vi "plc read string.vi"(8 "error in":errorcluster, 10 "Timeout (ms)":i32=1000, 11 "addr,tag":T1 {"DataSocket Reference"."OnStatusUpdated" format="%.0x"; "DataSocket Reference"."OnDataUpdated" format="%.0x"}) -> (0 "error out":errorcluster, 3 "Data":string)   [LabVIEW 2018]
uses:
  05.UserVI's/type defs/plc path and tag.ctl
  <vilib>/Platform/dataskt.llb/DataSocket Reference Type.ctl
  <vilib>/ethernetip/ethernetip.llb/EthernetIP Tag Read STRING.vi
  <vilib>/ethernetip/ethernetip.llb/EthernetIP Tag Read DINT.vi
  <vilib>/ethernetip/ethernetip.lvlib
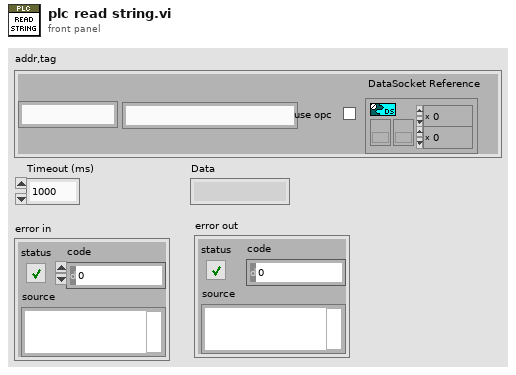
[diagram p1: front panel]
types:
  T1 = typedef "plc path and tag.ctl" = cluster{"Tag Name":string, "Network Path":string, "use opc":bool, "DataSocket Reference":T2}
  T2 = typedef "DataSocket Reference Type.ctl" = cluster{"CWDSLib._DCWDataSocket":refnum<k7>, "CWDSLib._DCWData":refnum<k7>, "OnDataUpdated":u32, "OnStatusUpdated":u32}
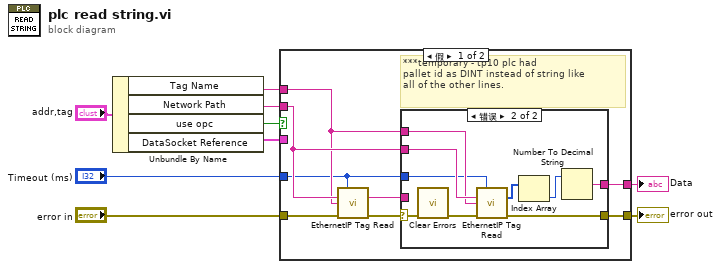
[diagram p0: block diagram]
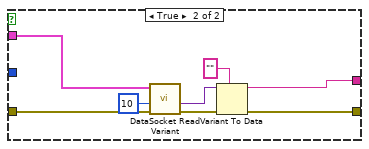
[diagram p3: hidden frame]
diagram:
  n1 = Unbundle By Name("addr,tag") -> ("Tag Name"=w4:string, "Network Path"=w5:string, "use opc"=w2:bool, "DataSocket Reference"=w1:T2)
  n2 = case shown="假" w2 {
    tunnel: "error in" -> [w17 w34]
    tunnel: [w14 w32] -> w7
    tunnel: [w13 w29] -> w6
    tunnel: w5 -> [w12 _]
    tunnel: w4 -> [w11 _]
    tunnel: "Timeout (ms)" -> [w10 _]
    tunnel: w1 -> [_ w35]
    frame False {
      # "***temporary - tp10 plc had\npallet id as DINT instead of string like\nall of the other lines."
      n3 = call-poly <vilib>:"EthernetIP Tag Read.vi"("Timeout (ms)"=w10, "Network Path"=w12, "Tag Name"=w11, "error in"=w17) -> ("Data"=w15:string, "error out"=w16:errorcluster)  [unwired: 9 in, 1 out]
      n4 = case shown="错误" w16 {
        selector: w16 -> [w18 w22]
        tunnel: [w19 w25] -> w13
        tunnel: w15 -> [w19 _]
        tunnel: w12 -> [_ w28]
        tunnel: w11 -> [_ w27]
        tunnel: [w18 w23] -> w14
        tunnel: w10 -> [_ w20]
        frame No Error {
        }
        frame Error {
          n5 = call <vilib>:"Clear Errors.vi"("error in (no error)"=w22) -> ("error out"=w21:errorcluster)  [unwired: 5 in, 1 out]
          n6 = call-poly <vilib>:"EthernetIP Tag Read.vi"("Timeout (ms)"=w20, "Network Path"=w28, "Tag Name"=w27, "error in"=w21) -> ("Data"=w26:i32[], "error out"=w23:errorcluster)  [unwired: 9 in, 1 out]
          n7 = Index Array(array=w26) -> (element=w24:i32)  [unwired: 1 in]
          n8 = Number To Decimal String(number=w24) -> (decimal integer string=w25:string)  [unwired: 1 in]
        }
      }
    }
    frame True {
      n9 = call <vilib>:"DataSocket Read Variant.vi"("error in (no error)"=w34, "Timeout (1000 ms)"=10, "DataSocket Reference In"=w35) -> ("error out"=w33:errorcluster, "Data"=w31:variant)  [unwired: 2 in, 3 out]
      n10 = Variant To Data(error in=w33, type="", Variant=w31) -> (data=w29:string, error out=w32:errorcluster)
    }
  }
  "Data" <- w6
  "error out" <- w7
